vi "Problem2.6.vi"() -> ()   [LabVIEW 2019]
panel:
  out "Distance":dbl
  out "Elapsed Time (s)":dbl
  out "Waveform Chart":dbl(graph)
  out "Speed":dbl
  in  "Distance":dbl(slide) scale=0.0..100.0
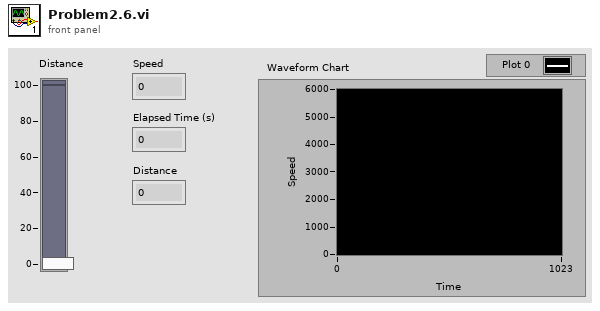
[diagram p1: front panel]
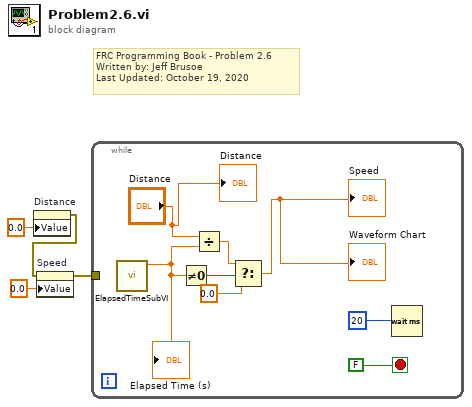
[diagram p0: block diagram]
diagram:
  # "FRC Programming Book - Problem 2.6\nWritten by: Jeff Brusoe\nLast Updated: October 19, 2020"
  n1 = property on="Distance" class="Slide (strict)"("Value"=0.0 ("Distance")) -> (error out=w2:errorcluster)  [unwired: 2 in, 1 out]
  n2 = property on="Speed" class="DigNum (strict)"(error in=w2, "Value"=0.0 ("Speed")) -> (error out=w1:errorcluster)  [unwired: 1 in, 1 out]
  n3 = while {
    tunnel: w1 -> [_]
    stop <- FALSE stop-if-true
    n4 = call "ElapsedTimeSubVI.vi"() -> ("Elapsed Time (s)"=w8:dbl)  [unwired: 11 in]
    "Elapsed Time (s)" <- w8
    n5 = Not Equal To 0?(x=w8) -> (x != 0?=w11:bool)
    n6 = Divide(x="Distance", y=w8) -> (x/y=w9:dbl)
    n7 = Select(t=w9, s=w11, f=0.0) -> (s? t:f=→"Waveform Chart" →"Speed":dbl)
    n8 = Wait (ms)(milliseconds to wait=u32 20) -> ()  [unwired: 1 out]
    "Distance" <- "Distance"
  }
